vi "GetDevInfo.vi"() -> (0 "Calibration Coefficients":string, 1 "Serial":string="HR1 3.0 c.N 0140")   [LabVIEW 2022 SP3]
uses:
  adcDLL_0001.dll
panel:
  out "Calibration Coefficients":u8[](array[numeric])
  out "Output Report":u8[](array[numeric])
  out "initialized array":u8[](array[numeric])
  in  "MaxExposure_seconds 2":u32
  in  "TotPixels 2":u32
  in  "DevDet_in":i32
  out "MaxExposure_seconds":u32
  out "TotPixels":u32
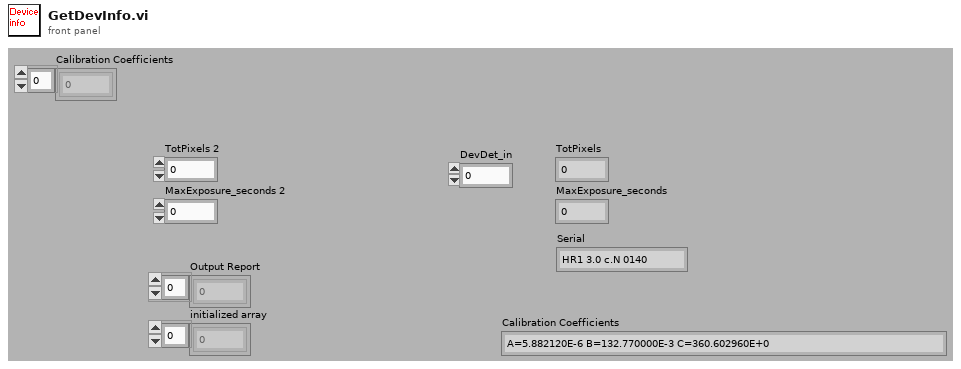
[diagram p1: front panel]
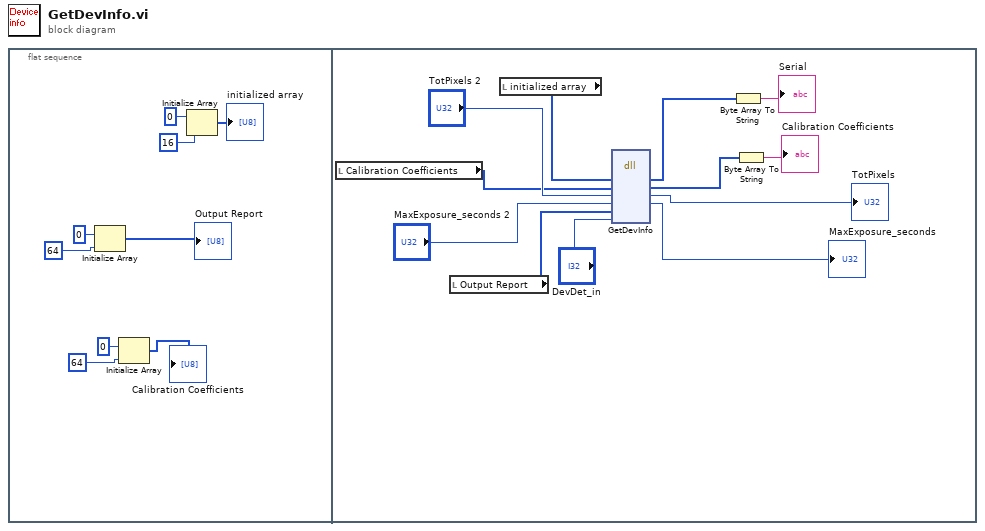
[diagram p0: block diagram]
diagram:
  n1 = flat-sequence {
    frame #0 {
      n2 = Initialize Array(u8 0 ("element"), 64 ("dimension size")) -> (→"Output Report":u8[])
      n3 = Initialize Array(u8 0 ("element"), 64 ("dimension size")) -> (→"Calibration Coefficients":u8[])
      n4 = Initialize Array(u8 0 ("element"), 16 ("dimension size")) -> (→"initialized array":u8[])
    }
    frame #1 {
      n5 = local read "Calibration Coefficients"() -> (w12:u8[])
      n6 = local read "Output Report"() -> (w21:u8[])
      n7 = local read "initialized array"() -> (w20:u8[])
      n8 = dll-call lib="D:/LabVIEWSuite_64_OS/Spectrometers/ASEQ LR1/adcDLL_0001.dll" fn="GetDevInfo"("Serial"=w20, "Calibration Coefficients"=w12, "TotPixels"="TotPixels 2", "MaxExposure_seconds"="MaxExposure_seconds 2", "Output Raport"=w21, "DevDet"="DevDet_in") -> ("Serial"=w14:u8[], "Calibration Coefficients"=w11:u8[], "TotPixels"=→"TotPixels":u32, "MaxExposure_seconds"=→"MaxExposure_seconds":u32)  [unwired: 6 in, 2 out]
      n9 = Byte Array To String(unsigned byte array=w14) -> (string=→"Serial":string)
      n10 = Byte Array To String(unsigned byte array=w11) -> (string=→"Calibration Coefficients":string)
    }
  }
